vi "test_RemoteDCPowerSession_CallCloseMeasurementLinkSessionWithDetachBehavior_RemoteSessionDetached.vi"(8 "error in":errorcluster) -> (0 "error out":errorcluster, 2 "result":string, 3 "pass":bool)   [LabVIEW 2020, in "MeasurementServerTests.lvlib"]
uses:
  MeasurementServerTests.lvlib
  Runtime/MeasurementLink niDCPower/Instrument/Session Factory.lvclass
  Runtime/MeasurementLink Instrument/IInstrument/Initialize and Close Session Behavior.ctl
  Runtime/MeasurementLink Instrument/IInstrument/ISession Factory.lvclass
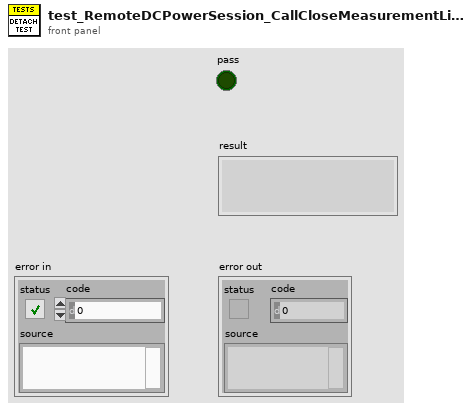
[diagram p1: front panel]
types:
  T1 = typedef "MeasurementLink Instrument.lvlib/ISession Factory.lvclass/Remote Connection Options.ctl" = cluster{"session name":string, "address":string, "port":u32}
  T2 = typedef "MeasurementLink Instrument.lvlib/ISession Factory.lvclass/Initialize and Close Session Behavior.ctl" = enum16{"Initialize and Close", "Attach and Detach", "Initialize and Detach", "Attach and Close"}
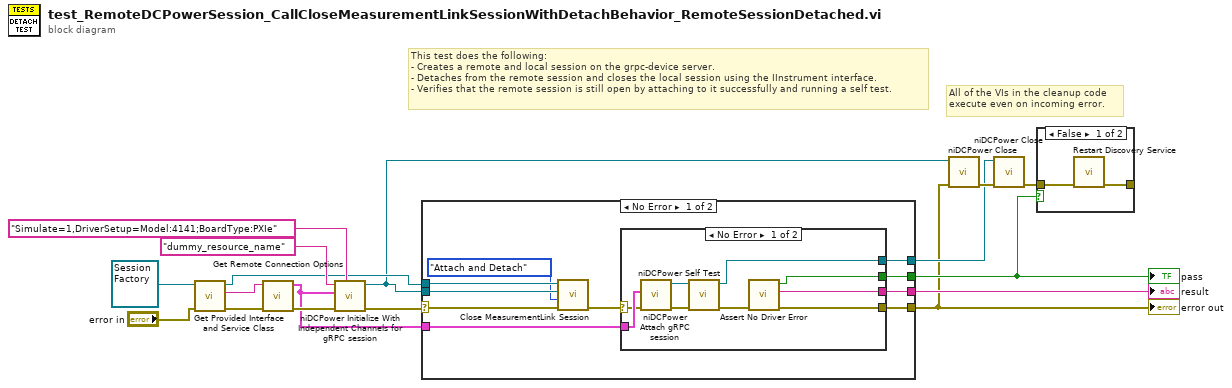
[diagram p0: block diagram]
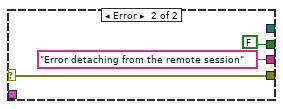
[diagram p2: hidden frame]
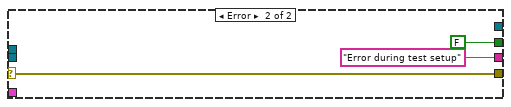
[diagram p3: hidden frame]
diagram:
  # "All of the VIs in the cleanup code\nexecute even on incoming error."
  # "This test does the following:\n- Creates a remote and local session on the grpc-device server.\n- Detaches from the remote session and closes the local session using the IInstrument interface.\n- Verifies that the remote session is still open by attaching to it successfully and running a self test."
  n1 = call-dynamic "Get Provided Interface and Service Class.vi"("error in"="error in", "instrument in"=refnum<class "Session Factory.lvclass"> refnum ("MeasurementLink niDCPower.lvlib:Instrument.lvclass")) -> ("error out"=w14:errorcluster, "provided interface"=w13:string, "instrument out"=w9:refnum<class "Session Factory.lvclass">)  [unwired: 6 in, 1 out]
  n2 = call "Get Remote Connection Options.vi"("error in"=w14, "provided interface"=w13) -> ("error out"=w16:errorcluster, "remote connection options"=w8:T1)  [unwired: 8 in]
  n3 = call <instrlib>:"niDCPower Initialize With Independent Channels for gRPC session.vi"("option string"="Simulate=1,DriverSetup=Model:4141;BoardType:PXIe", "error in (no error)"=w16, "gRPC options"=w8, "resource name"="dummy_resource_name") -> ("error out"=w10:errorcluster, "instrument handle out"=w3:refnum<k15>)  [unwired: 6 in]
  n4 = case shown="No Error" w10 {
    selector: w10 -> [w27 w41]
    tunnel: w9 -> [w26 _]
    tunnel: w3 -> [w25 _]
    tunnel: w8 -> [w24 _]
    tunnel: [w22 w41] -> w1
    tunnel: [w21 FALSE] -> w4
    tunnel: [w20 "Error during test setup" ("f")] -> w7
    tunnel: [w18 _] -> w2
    frame No Error {
      n5 = call-dynamic "Close MeasurementLink Session.vi"("error in"=w27, "initialize and close session behavior"=Initialize_and_Close_Session_Behavior."Attach and Detach", "session in"=w25, "instrument in"=w26) -> ("error out"=w23:errorcluster)  [unwired: 7 in]
      n6 = case shown="No Error" w23 {
        selector: w23 -> [w35 w37]
        tunnel: w24 -> [w36 _]
        tunnel: [w30 w37] -> w22
        tunnel: [w28 FALSE] -> w21
        tunnel: [w29 "Error detaching from the remote session" ("f")] -> w20
        tunnel: [w32 _] -> w18
        frame No Error {
          n7 = call <instrlib>:"niDCPower Attach gRPC session.vi"("error in (no error)"=w35, "gRPC options"=w36) -> ("error out"=w33:errorcluster, "instrument handle out"=w34:refnum<k15>)  [unwired: 8 in]
          n8 = call <instrlib>:"niDCPower Self Test.vi"("error in (no error)"=w33, "instrument handle"=w34) -> ("error out"=w31:errorcluster, "instrument handle out"=w32:refnum<k15>)  [unwired: 6 in, 2 out]
          n9 = call "Assert No Driver Error.vi"("error in"=w31) -> ("error out"=w30:errorcluster, "result"=w29:string, "pass?"=w28:bool)  [unwired: 8 in]
        }
        frame Error {
        }
      }
    }
    frame Error {
    }
  }
  "error out" <- w1
  "pass" <- w4
  "result" <- w7
  n10 = call <instrlib>:"niDCPower Close.vi"("error in (no error)"=w1, "instrument handle"=w3) -> ("error out"=w6:errorcluster)  [unwired: 9 in]
  n11 = call <instrlib>:"niDCPower Close.vi"("error in (no error)"=w6, "instrument handle"=w2) -> ("error out"=w5:errorcluster)  [unwired: 9 in]
  n12 = case shown="False" w4 {
    tunnel: [w44 _] -> _
    tunnel: w5 -> [w43 _]
    frame False {
      n13 = call "Restart Discovery Service.vi"("error in"=w43) -> ("error out"=w44:errorcluster)  [unwired: 10 in]
    }
    frame True {
    }
  }
